vi "CalculateInterceptingPoint.vi"(0 "object in":refnum<class "WaitBallTrajSkill.lvclass">, 5 "error in (no error)":errorcluster) -> (14 "object out":refnum<class "WaitBallTrajSkill.lvclass">, 19 "error out":errorcluster)   [LabVIEW 2023, in "WaitBallTrajSkill.lvclass"]
uses:
  WaitBallTrajSkill.lvclass
  Ball_class/Ball.lvclass
  C:/Users/ebert/Documents/codes/SSL/repo/SSL_AI/Object_class/Object.lvclass
  Robot_class/Robot.lvclass
  Object_class/Object.lvclass/Object.ctl
  Ball_class/Ball.lvclass/Ball.ctl
  Object_class/Read position(x,y).vi
  Ball_class/Read v_x.vi
  Ball_class/Read v_y.vi
panel:
  in  "Robot":refnum<class "Robot.lvclass">
  out "Intercepting Point":dbl[](array[numeric])
  in  "Ball":refnum<class "Ball.lvclass">
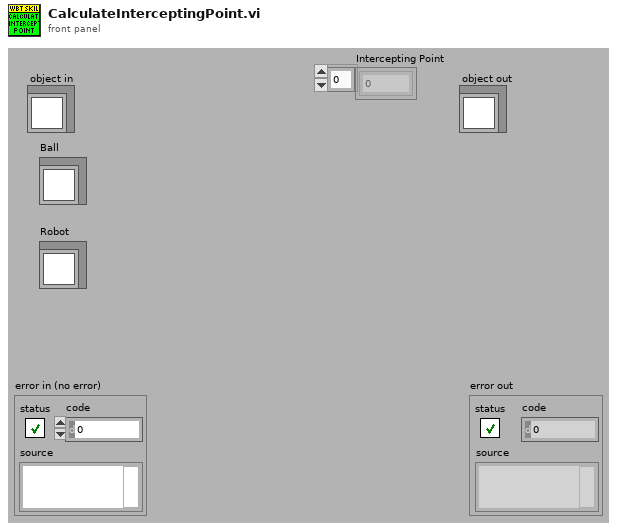
[diagram p1: front panel]
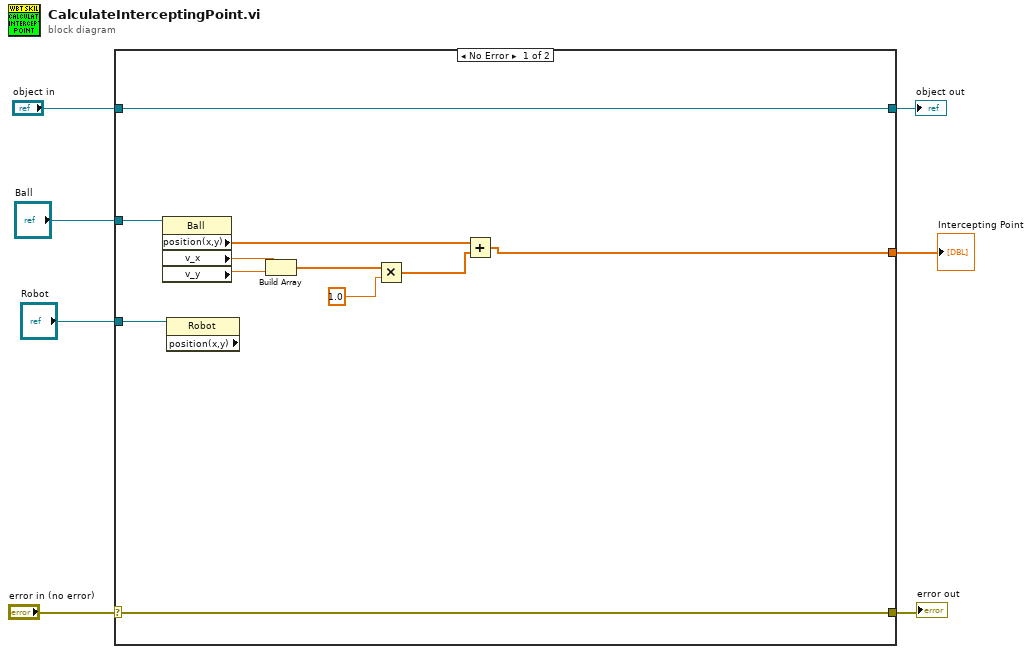
[diagram p0: block diagram]
diagram:
  n1 = case shown="No Error" "error in (no error)" {
    selector: "error in (no error)" -> [w17 w20]
    tunnel: [w17 w20] -> w6
    tunnel: [w18 w19] -> w4
    tunnel: "object in" -> [w18 w19]
    tunnel: "Ball" -> [w16 _]
    tunnel: [w10 _] -> w2
    tunnel: "Robot" -> [w9 _]
    frame No Error {
      n2 = property class="Ball"(reference=w16) -> ("position(x,y)"=w15:dbl[], "v_x"=w13:dbl, "v_y"=w12:dbl)  [unwired: 1 in, 2 out]
      n3 = property class="Robot" props=["position(x,y)"](reference=w9) -> ()  [unwired: 1 in, 3 out]
      n4 = Build Array(w13, w12) -> (w14:dbl[])
      n5 = Multiply(x=w14, y=1.0) -> (x*y=w11:dbl[])
      n6 = Add(x=w15, y=w11) -> (x+y=w10:dbl[])
    }
    frame Error {
    }
  }
  "error out" <- w6
  "object out" <- w4
  "Intercepting Point" <- w2
